vi "Rohde & Schwarz VNA Set Sweep Time.vi"(6 "Channel":i8=1 min=1 max=99 step=1, 7 "Rohde & Schwarz VNA":T1, 8 "error in (no error)":errorcluster, 10 "Sweep Time, s (-1: Auto)":dbl=-1.0, 11 "VISA Resource Name":refnum<visa-resource-name>) -> (0 "error out":errorcluster, 3 "dup VISA Resource Name":refnum<visa-resource-name>)   [LabVIEW 2011]
doc: "This Vi for the HP8753B Network Analyzer is used to set averaging, smoothing, and the IF bandwidth."
uses:
  TypeDefs/Rohde & Schwarz VNA Instrument Info.ctl
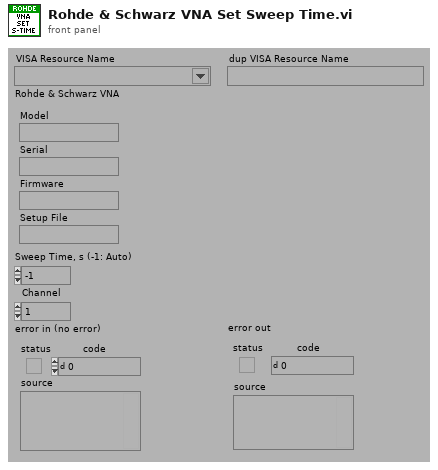
[diagram p1: front panel]
types:
  T1 = typedef "Rohde & Schwarz VNA Instrument Info.ctl" = cluster{"Model":string, "Serial":string, "Firmware":string, "Setup File":string}
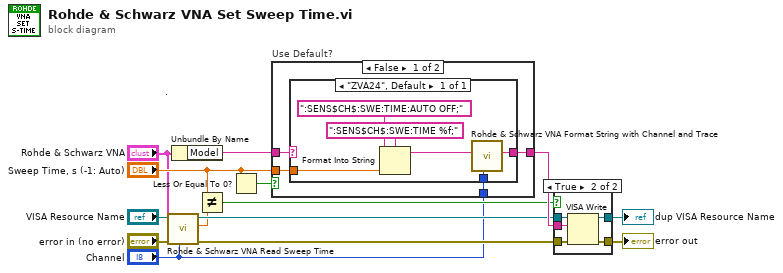
[diagram p0: block diagram]
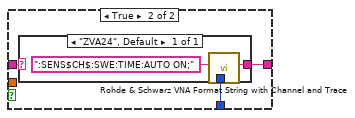
[diagram p3: hidden frame]
diagram:
  # "."
  n1 = call "Rohde & Schwarz VNA Read Sweep Time.vi"("Channel"="Channel", "Rohde & Schwarz VNA"="Rohde & Schwarz VNA", "error in (no error)"="error in (no error)", "VISA Resource Name"="VISA Resource Name") -> ("error out"=w7:errorcluster, "Sweep Time, s"=w6:dbl, "dup VISA Resource Name"=w8:refnum<visa-resource-name>)  [unwired: 5 out]
  n2 = Unbundle By Name("Rohde & Schwarz VNA") -> ("Model"=w1:string)
  n3 = Not Equal?(x="Sweep Time, s (-1: Auto)", y=w6) -> (x != y?=w4:bool)
  n4 = Less Or Equal To 0?(x="Sweep Time, s (-1: Auto)") -> (x <= 0?=w12:bool)
  n5 = case "Use Default?" shown="False" w12 {
    tunnel: "Sweep Time, s (-1: Auto)" -> [w18 _]
    tunnel: [w17 w27] -> w11
    tunnel: w1 -> [w16 w26]
    tunnel: "Channel" -> [w15 w25]
    frame False {
      n6 = case shown="\"ZVA24\", Default" w16 {
        tunnel: w18 -> [w23]
        tunnel: [w20] -> w17
        tunnel: w15 -> [w19]
        frame "ZVA24", Default {
          n7 = Format Into String(format string=":SENS$CH$:SWE:TIME %f;", initial string=":SENS$CH$:SWE:TIME:AUTO OFF;", w23) -> (resulting string=w21:string)  [unwired: 1 in, 1 out]
          n8 = call "Rohde & Schwarz VNA Format String with Channel and Trace.vi"("Channel"=w19, "String"=w21) -> ("String Out"=w20:string)  [unwired: 1 in, 6 out]
        }
      }
    }
    frame True {
      n9 = case shown="\"ZVA24\", Default" w26 {
        tunnel: [w29] -> w27
        tunnel: w25 -> [w28]
        frame "ZVA24", Default {
          n10 = call "Rohde & Schwarz VNA Format String with Channel and Trace.vi"("Channel"=w28, "String"=":SENS$CH$:SWE:TIME:AUTO ON;") -> ("String Out"=w29:string)  [unwired: 1 in, 6 out]
        }
      }
    }
  }
  n11 = case shown="True" w4 {
    tunnel: [w31 w37] -> w14
    tunnel: [w32 w36] -> w13
    tunnel: w11 -> [_ w35]
    tunnel: w8 -> [w32 w34]
    tunnel: w7 -> [w31 w33]
    frame False {
    }
    frame True {
      n12 = VISA Write(VISA resource name=w34, write buffer=w35, error in (no error)=w33) -> (VISA resource name out=w36:refnum<visa-resource-name>, error out=w37:errorcluster)  [unwired: 1 out]
    }
  }
  "error out" <- w14
  "dup VISA Resource Name" <- w13
